vi "Get Macro by Name.vi"(8 "error in (no error)":errorcluster, 10 "Macro Name":string, 11 "Motions in":refnum<class "Motions.lvclass">) -> (0 "error out":errorcluster, 1 "found":bool, 2 "TriggerAction Q.lvclass":refnum<class "TriggerAction Q.lvclass">, 3 "Motions out":refnum<class "Motions.lvclass">)   [LabVIEW 2016, in "Hardware.lvlib" / "Motions.lvlib" / "Motions.lvclass"]
uses:
  <userlib>/Common Components/Hardware/Abstract System/Motions/Motions/Motions.lvclass
  <userlib>/Common Components/TriggerAction Q/TriggerAction Q/TriggerAction Q.lvclass
  <userlib>/Common Components/Hardware/Abstract System/Motions/Motions/Motions.lvclass/Motions.ctl
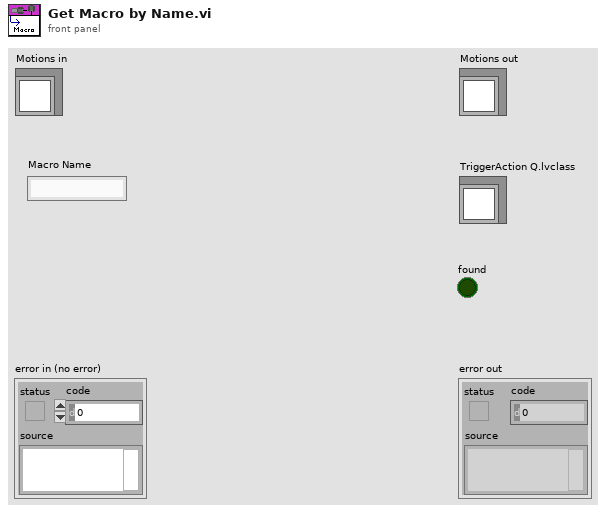
[diagram p1: front panel]
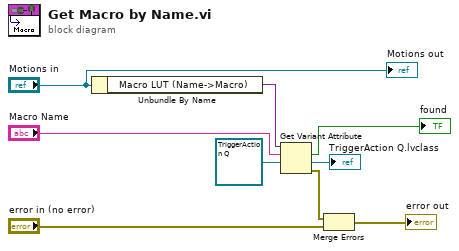
[diagram p0: block diagram]
diagram:
  n1 = Unbundle By Name("Motions in") -> ("Macro LUT (Name->Macro)"=w7:variant)
  n2 = Get Variant Attribute(Variant=w7, name="Macro Name", default value (empty Variant)=refnum<class "TriggerAction Q.lvclass"> refnum ("TriggerAction Q.lvclass")) -> (found=→"found":bool, value=→"TriggerAction Q.lvclass":refnum<class "TriggerAction Q.lvclass">, error out=w3:errorcluster)  [unwired: 1 in, 1 out]
  n3 = Merge Errors(w3, "error in (no error)") -> (→"error out":errorcluster)
  "Motions out" <- "Motions in"
